vi "defer panel updates VIref step1.vi"(8 "error in (no error)":errorcluster, 11 "VI reference":refnum<vi>) -> (0 "error out":errorcluster, 3 "Refs":T1)   [LabVIEW 2019, in "Defer Panel Updates BVV.lvlib"]
uses:
  Defer Panel Updates BVV.lvlib
  defer panel updates data.ctl
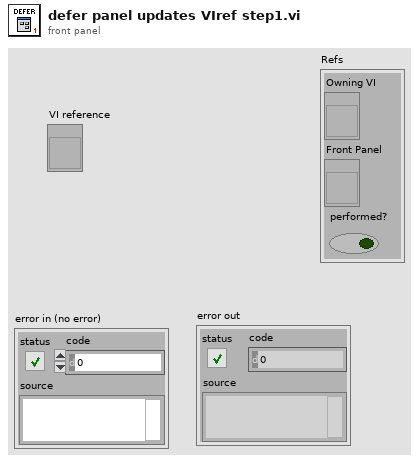
[diagram p1: front panel]
types:
  T1 = typedef "Defer Panel Updates BVV.lvlib/defer panel updates data.ctl" = cluster{"Owning VI":refnum<vi>, "Front Panel":refnum<vi>, "performed?":bool}
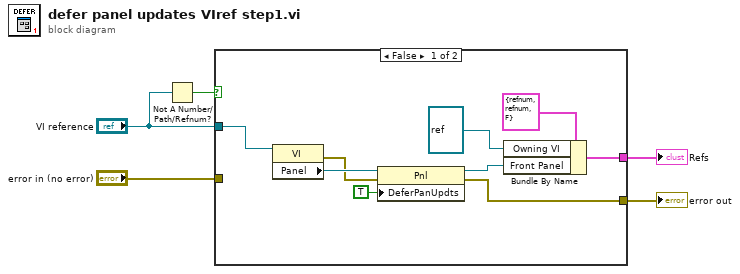
[diagram p0: block diagram]
diagram:
  n1 = Not A Number/Path/Refnum?(number/path/refnum="VI reference") -> (NaN/Path/Refnum?=w5:bool)
  n2 = case shown="False" w5 {
    tunnel: "VI reference" -> [w7 _]
    tunnel: "error in (no error)" -> [_ w15]
    tunnel: [w9 w15] -> w3
    tunnel: [w8 _] -> w2
    frame False {
      n3 = property class="VI"(reference=w7) -> (error out=w12:errorcluster, "Panel"=w14:refnum<vi>)  [unwired: 1 in, 1 out]
      n4 = property class="Pnl"(reference=w14, error in=w12, "DeferPanUpdts"=TRUE ("Defer Panel Updates")) -> (reference out=w10:refnum<vi>, error out=w9:errorcluster)
      n5 = Bundle By Name(cluster=T1 {"Owning VI"=refnum, "Front Panel"=refnum, "performed?"=FALSE}, "Owning VI"=refnum<vi> refnum, "Front Panel"=w10) -> (w8:T1)
    }
    frame True {
    }
  }
  "error out" <- w3
  "Refs" <- w2
